vi "Handle.vi"(8 "error in (no error)":errorcluster, 10 "Zero Timeout Message Handler in":refnum<class "Zero Timeout Message Handler.lvclass">, 11 "Message in":refnum<class "Stop Polling Msg.lvclass">) -> (0 "error out":errorcluster, 2 "Zero Timeout Message Handler out":refnum<class "Zero Timeout Message Handler.lvclass">)   [LabVIEW 2024, in "Zero Timeout Message Handler.lvlib" / "Stop Polling Msg.lvclass"]
uses:
  Stop Polling Msg.lvclass
  Zero Timeout Message Handler/Zero Timeout Message Handler.lvclass
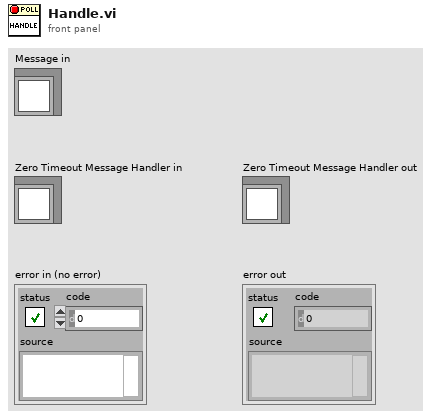
[diagram p1: front panel]
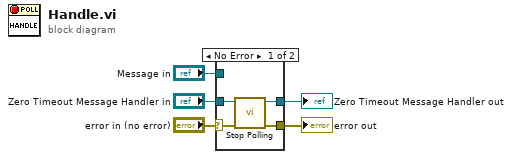
[diagram p0: block diagram]
diagram:
  n1 = case shown="No Error" "error in (no error)" {
    selector: "error in (no error)" -> [w6 w11]
    tunnel: [w7 w11] -> w4
    tunnel: [w8 w10] -> w3
    tunnel: "Zero Timeout Message Handler in" -> [w9 w10]
    tunnel: "Message in" -> [_ _]
    frame No Error {
      n2 = call-dynamic "Stop Polling.vi"("error in (no error)"=w6, "Zero Timeout Message Handler in"=w9) -> ("error out"=w7:errorcluster, "Zero Timeout Message Handler out"=w8:refnum<class "Zero Timeout Message Handler.lvclass">)  [unwired: 8 in]
    }
    frame Error {
    }
  }
  "error out" <- w4
  "Zero Timeout Message Handler out" <- w3
